vi "set start node.vi"(8 "error in (no error)":errorcluster, 10 "start node path":string, 11 "alias-tree in":refnum<class "alias-tree.lvclass">) -> (0 "error out":errorcluster, 3 "alias-tree out":refnum<class "alias-tree.lvclass">)   [LabVIEW 2017, in "vs-tree-utility.lvlib" / "alias-tree.lvclass"]
uses:
  alias-tree.lvclass
  alias-tree.lvclass/alias-tree.ctl
  NationalInstruments.VeriStand.SystemStorageUI
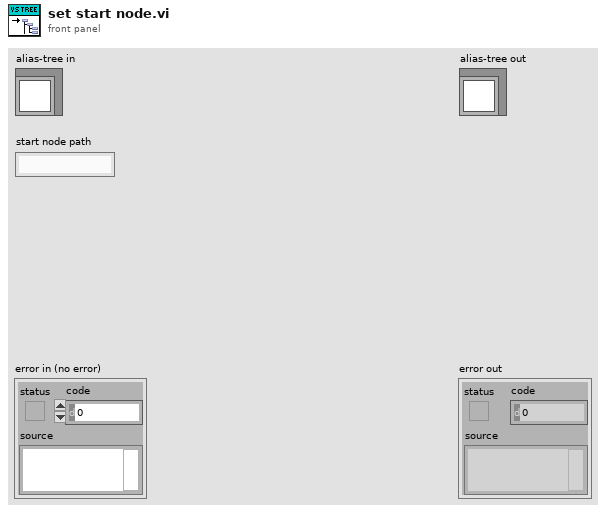
[diagram p1: front panel]
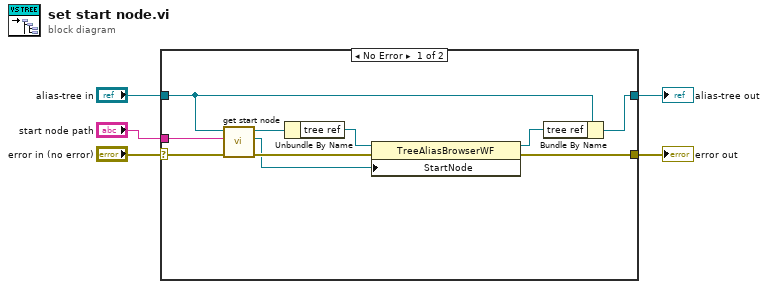
[diagram p0: block diagram]
diagram:
  n1 = case shown="No Error" "error in (no error)" {
    selector: "error in (no error)" -> [w15 w16]
    tunnel: [w8 w17] -> w4
    tunnel: "alias-tree in" -> [w9 w17]
    tunnel: [w7 w16] -> w2
    tunnel: "start node path" -> [w14 _]
    frame No Error {
      n2 = call-dynamic "get start node.vi"("error in (no error)"=w15, "start node path (root)"=w14, "abstract-tree in"=w9) -> ("error out"=w12:errorcluster, "start node"=w10:refnum<k24>, "abstract-tree out"=w13:refnum<class "alias-tree.lvclass">)  [unwired: 6 in]
      n3 = Unbundle By Name(w13) -> ("tree ref"=w11:refnum<k24>)
      n4 = property class="TreeAliasBrowserWF"(reference=w11, error in=w12, "StartNode"=w10) -> (reference out=w6:refnum<k24>, error out=w7:errorcluster)
      n5 = Bundle By Name(cluster=w9, "tree ref"=w6) -> (w8:refnum<class "alias-tree.lvclass">)
    }
    frame Error {
    }
  }
  "error out" <- w2
  "alias-tree out" <- w4
